vi "SetLimit.vi"(8 "error in":errorcluster, 10 "Limit":refnum<class "MeasureLimit.lvclass">, 11 "Measure in":refnum<class "Measure.lvclass">) -> (0 "error out":errorcluster, 3 "Measure out":refnum<class "Measure.lvclass">)   [LabVIEW 2021, in "ProligentXMLGenerator.lvlib" / "Measure.lvclass"]
doc: "Defines the date when the measure was acquired.\n\nThis vaule is restricted to \"1900-01-01T00:00:00Z\" -\"2100-01-01T00:00:00Z\""
uses:
  Measure.lvclass
  Measure.lvclass/Measure.ctl
  MeasureLimit/MeasureLimit.lvclass
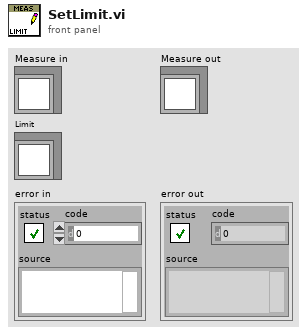
[diagram p1: front panel]
types:
  T1 = typedef "ProligentXMLGenerator.lvlib/Measure.lvclass/Data.ctl" = cluster{"Name":string, "Type":refnum<class "MeasureKind.lvclass">, "Precision":refnum<class "UnsignedByte.lvclass">, "Limit":refnum<class "MeasureLimit.lvclass">, "Characteristics":refnum<class "Characteristic.lvclass">[], "FailureReferences":refnum<class "FailureReference.lvclass">[], "CustomData":refnum<class "CustomData.lvclass">, "MeasureId":refnum<class "Guid.lvclass">, "MeasureTime":refnum<class "DateTime.lvclass">, "Comments":refnum<class "NonNullableString_TruncateAt_255.lvclass">, "Unit":refnum<class "NonEmptyString_30.lvclass">, "Symbol":refnum<class "NonEmptyString_20.lvclass">, "MeasureExecutionStatus":refnum<class "ExecutionStatus.lvclass">}
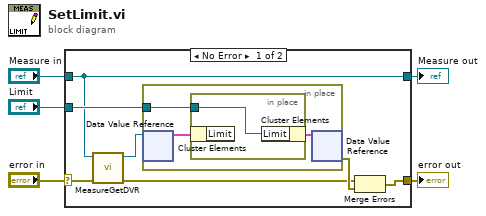
[diagram p0: block diagram]
diagram:
  n1 = case shown="No Error" "error in" {
    selector: "error in" -> [w10 w17]
    tunnel: "Measure in" -> [w7 w18]
    tunnel: [w9 w17] -> w3
    tunnel: "Limit" -> [w8 _]
    tunnel: [w7 w18] -> w1
    frame No Error {
      n2 = call "MeasureGetDVR.vi"("error in"=w10, "Measure"=w7) -> ("error out"=w6:errorcluster, "DVRReference"=w11:refnum<data-value>)  [unwired: 8 in]
      n3 = in-place "In Place Element Structure" {
        in-place-border: w8 -> [w15]
        n4 = in-place-dvr #1(w11) -> (w14:T1)  [unwired: 1 out]
        n5 = in-place "In Place Element Structure" {
          in-place-border: w15 -> [w16]
          n6 = in-place-cluster #2(w14) -> ()  [unwired: 1 out]
          n7 = in-place-cluster #2("Limit"=w16) -> (w13:T1)
        }
        n8 = in-place-dvr #1(w13) -> (w12:errorcluster)  [unwired: 1 out]
      }
      n9 = Merge Errors(w6, w12) -> (w9:errorcluster)
    }
    frame Error {
    }
  }
  "error out" <- w3
  "Measure out" <- w1
